vi "load calibration profile data.vi"(8 "error in":errorcluster, 11 "Path":path) -> (0 "error out":errorcluster, 1 "Calibration params":T1[](array[typedef]), 2 "Image names":string[](array[string]), 3 "Image Array refs":T3[](array[typedef]), 4 "Scanning params":T2[](array[typedef]), 5 "Sr No.":i32[](array[numeric]))   [LabVIEW 2020]
uses:
  <vilib>/vision/Image Controls.llb/IMAQ Image.ctl
  TypeDefs/Current Imaging Parameters.ctl
  TypeDefs/Current Calibration Parameters.ctl
panel:
  out "number":dbl[][](array[numeric])
  out "array w/ subset deleted":string[][](array[string])
  out "Column Headers":string[][](array[string])
  out "Data":string[][](array[string])
  out "name":string
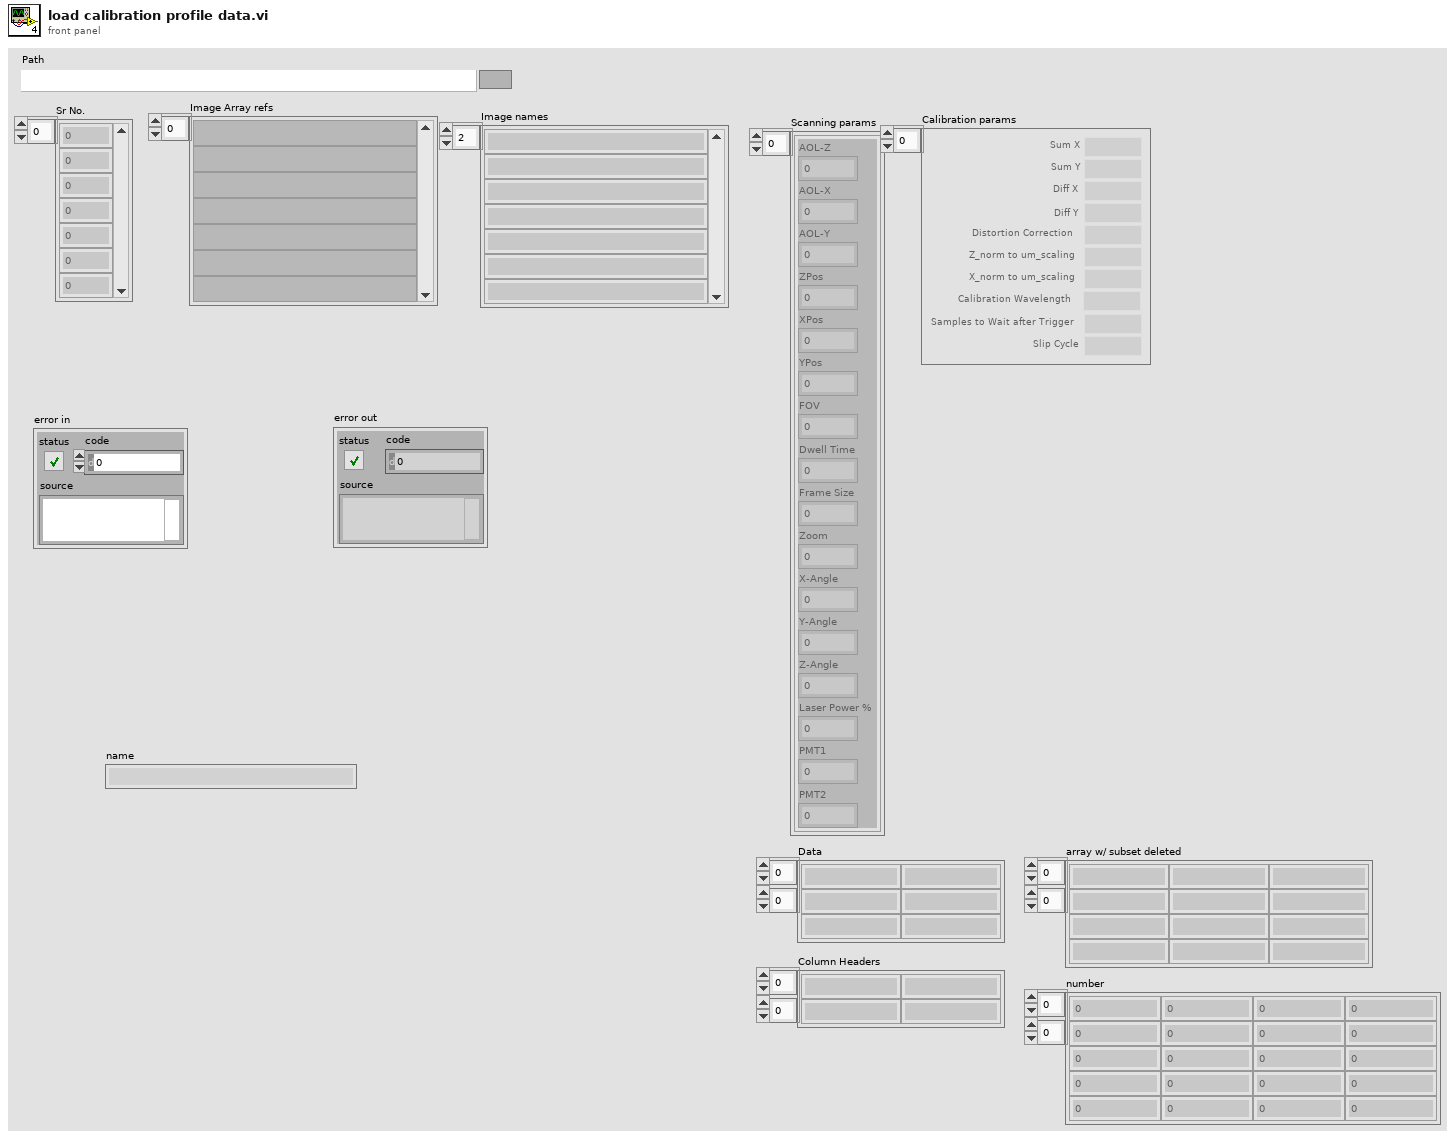
[diagram p1: front panel]
types:
  T1 = typedef "Current Calibration Parameters.ctl" = cluster{"Sum X":dbl, "Sum Y":dbl, "Diff X":dbl, "Diff Y":dbl, "Distortion Correction":dbl, "Z_norm to um_scaling":dbl, "X_norm to um_scaling":dbl, "Samples to Wait after Trigger":dbl, "Slip Cycle":dbl, "Calibration Wavelength":dbl}
  T2 = typedef "Current Imaging Parameters.ctl" = cluster{"AOL-Z":dbl, "AOL-X":dbl, "AOL-Y":dbl, "ZPos":dbl, "XPos":dbl, "YPos":dbl, "FOV":dbl, "Dwell Time":dbl, "Frame Size":dbl, "Zoom":dbl, "X-Angle":dbl, "Y-Angle":dbl, "Z-Angle":dbl, "Laser Power %":dbl, "PMT1":dbl, "PMT2":dbl}
  T3 = typedef "IMAQ Image.ctl" = refnum<image>
  T4 = typedef "Fixed strings.ctl" = cluster{"ROI file name":string, "Normalised ROI file name":string, "Zplane Pockels values file name":string, "Functional data folder name":string, "Experiment Header file name":string, "Z-stack images folder name":string, "Groups setup rel. path":string, "Groups text file rel. path":string, "TDMS files folder name (F.img)":string, "TDMS files folder name (V.acq)":string, "TDMS files folder name (Pl.acq)":string, "Cycle rel times sequence file":string, "Dynamically called VIs folder name":string, "Time Series folder base name":string, "Parameter Sweep":string, "Calibration Profile Images":string}
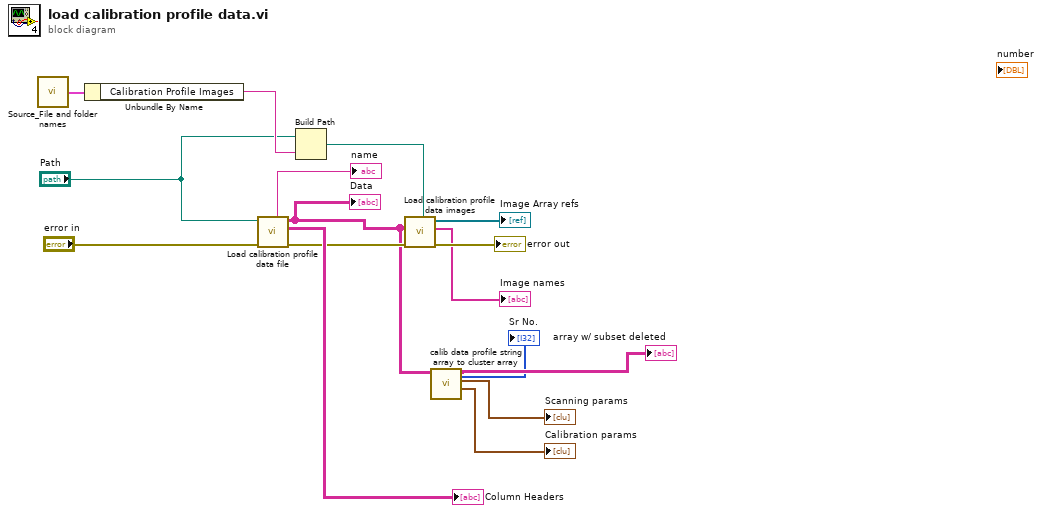
[diagram p0: block diagram]
diagram:
  n1 = call "Source_File and folder names.vi"() -> ("Fixed strings"=w16:T4)  [unwired: 1 in]
  n2 = Unbundle By Name(w16) -> ("Calibration Profile Images"=w15:string)
  n3 = call "Load calibration profile data file.vi"("error in (no error)"="error in", "Path"="Path") -> ("error out"=w7:errorcluster, "Column Headers"=→"Column Headers":string[][], "Data"=w5:string[][], "File Name"=→"name":string)  [unwired: 6 in]
  "Data" <- w5
  n4 = Build Path(base path="Path", name or relative path=w15) -> (appended path=w13:path)
  n5 = call "Load calibration profile data images.vi"("error in (no error)"=w7, "Array"=w5, "appended path"=w13) -> ("error out"=→"error out":errorcluster, "Image names"=→"Image names":string[], "Image Array refs"=→"Image Array refs":T3[])  [unwired: 6 in]
  n6 = call "calib data profile string array to cluster array.vi"("Data"=w5) -> ("Array 2"=→"Calibration params":T1[], "Array"=→"Scanning params":T2[], "array w/ subset deleted"=→"array w/ subset deleted":string[][], "Sr No."=→"Sr No.":i32[])  [unwired: 7 in]
